vi "Tester.vi"() -> ()   [LabVIEW 2020, in "Process Generation.lvlib" / "Process Generator.lvclass"]
uses:
  Process Generator.lvclass
  Process Generator.lvclass/Process Generator.ctl
  Framework/Process/Process.lvclass
panel:
  in  "Numeric":i32
  out "error out":errorcluster
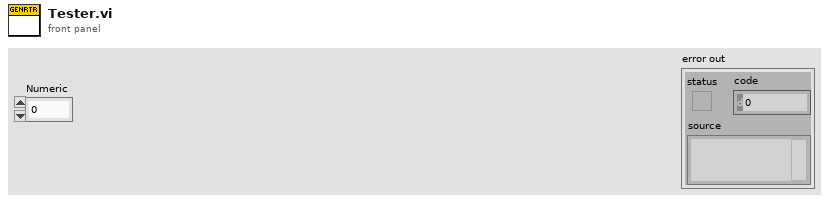
[diagram p1: front panel]
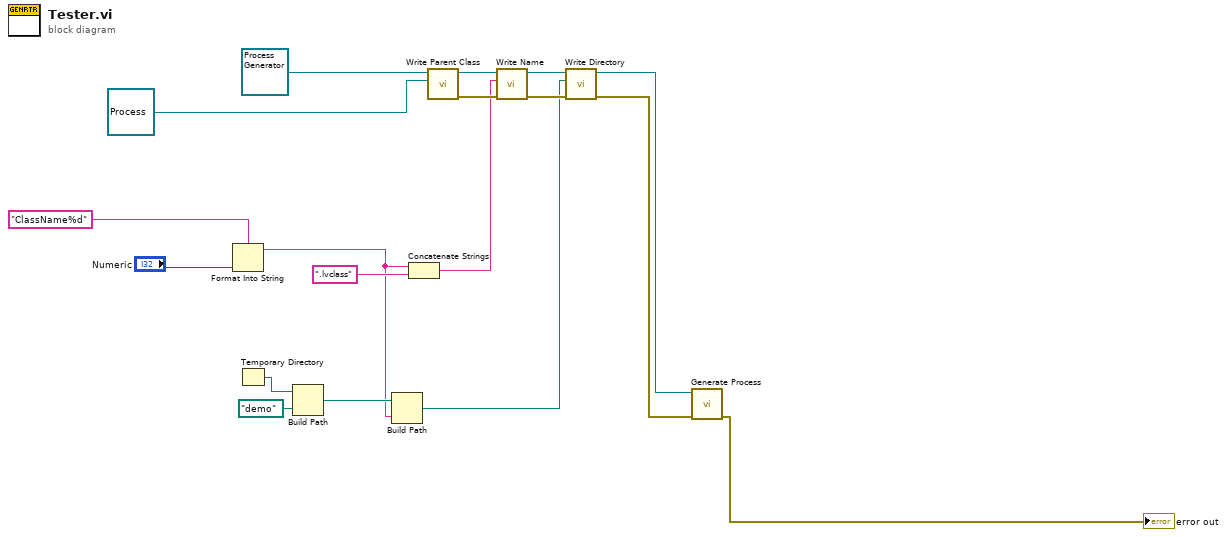
[diagram p0: block diagram]
diagram:
  n1 = Format Into String(format string="ClassName%d", "Numeric") -> (resulting string=w13:string)  [unwired: 2 in, 1 out]
  n2 = Temporary Directory() -> (w18:path)
  n3 = Build Path(base path=w18, name or relative path=path "demo") -> (appended path=w16:path)
  n4 = Build Path(base path=w16, name or relative path=w13) -> (appended path=w1:path)
  n5 = Concatenate Strings(w13, ".lvclass" ("string")) -> (w2:string)
  n6 = call "Write Parent Class.vi"("Parent Process"=refnum<class "Process.lvclass"> refnum ("Parent Class"), "Process Generator in"=refnum<class "Process Generator.lvclass"> refnum ("Process Generator In")) -> ("error out"=w5:errorcluster, "Process Generator out"=w6:refnum<class "Process Generator.lvclass">)  [unwired: 8 in]
  n7 = call "Write Name.vi"("error in (no error)"=w5, "Name"=w2, "Process Generator In"=w6) -> ("error out"=w7:errorcluster, "Process Generator Out"=w8:refnum<class "Process Generator.lvclass">)  [unwired: 7 in]
  n8 = call "Write Directory.vi"("error in (no error)"=w7, "Directory"=w1, "Process Generator in"=w8) -> ("error out"=w3:errorcluster, "Process Generator out"=w4:refnum<class "Process Generator.lvclass">)  [unwired: 7 in]
  n9 = call "Generate Process.vi"("error in (no error)"=w3, "Process Generator In"=w4) -> ("error out"=→"error out":errorcluster)  [unwired: 8 in, 1 out]
